vi "DEV Get Timestamp.vi"(9 "pTimestamp":u32, 10 "BusType":i8, 11 "DevHandle":i32) -> (1 "pTimestamp out":u32, 3 "function return":u8)   [LabVIEW 2010, in "usb_device.lvlib"]
doc: "unsigned char WINAPI DEV_GetTimestamp(int DevHandle,char BusType,unsigned int *pTimestamp);"
uses:
  usb_device.lvlib
  USB2XXX/trunk/USB2XXX/USB2XXX/vs2019/Release/USB2XXX.dll
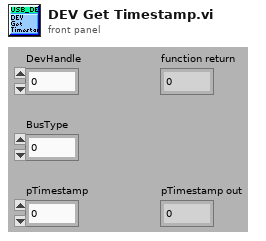
[diagram p1: front panel]
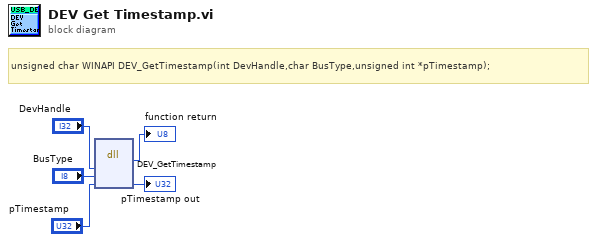
[diagram p0: block diagram]
diagram:
  # "unsigned char WINAPI DEV_GetTimestamp(int DevHandle,char BusType,unsigned int *pTimestamp);"
  n1 = dll-call lib="E:/Projects/USB2XXX/trunk/USB2XXX/USB2XXX/vs2019/Release/USB2XXX.*" fn="DEV_GetTimestamp"("DevHandle"="DevHandle", "BusType"="BusType", "pTimestamp"="pTimestamp") -> (→"function return":u8, "pTimestamp"=→"pTimestamp out":u32)  [unwired: 5 in, 2 out]
